vi "GD_GesamtKonz_EA_back_calc.vi"(7 "DoIt":bool, 8 "Einheit in String":string, 9 "höchste Konzentration Teilkomponente":dbl, 10 "Gesamtkonzentration":dbl, 11 "Stufentabelle (Eingang)":string[](array[string])) -> (3 "Sollwerte EA Tabelle (Ausgang)":string[](array[string]))   [LabVIEW 2020, in "Linearisierung v2.lvlib" / "Gasteiler.lvlib"]
uses:
  Gasteiler.lvlib
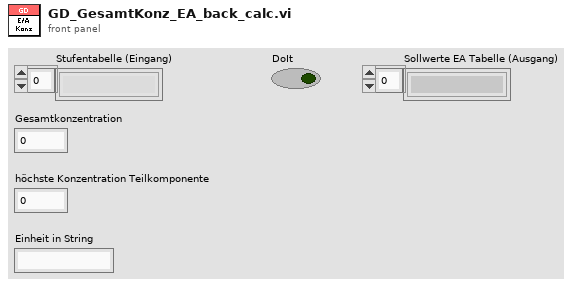
[diagram p1: front panel]
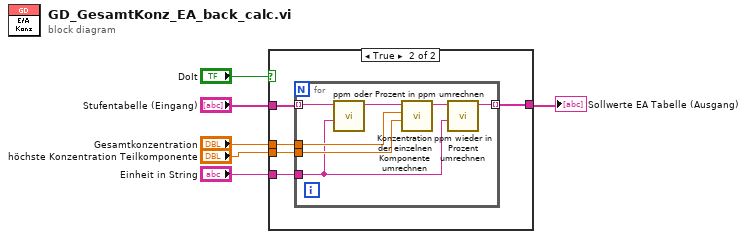
[diagram p0: block diagram]
diagram:
  n1 = case shown="True" "DoIt" {
    tunnel: "Stufentabelle (Eingang)" -> [w7 w12]
    tunnel: "Gesamtkonzentration" -> [_ w11]
    tunnel: "höchste Konzentration Teilkomponente" -> [_ w10]
    tunnel: "Einheit in String" -> [_ w9]
    tunnel: [w7 w8] -> w5
    frame False {
    }
    frame True {
      n2 = for {
        tunnel: w10 -> [w18]
        tunnel: w9 -> [w13]
        tunnel: w12 -> [w15] mode=indexing
        tunnel: w11 -> [w17]
        tunnel: [w16] -> w8 mode=indexing
        n3 = call "ppm oder Prozent in ppm umrechnen.vi"("Einheit"=w13, "Werteingang"=w15) -> ("Wertausgang"=w14:string)  [unwired: 9 in]
        n4 = call "Konzentration der einzelnen Komponente umrechnen.vi"("Teilkonzentration"=w18, "Gesamtkonzentration"=w17, "Werteingang"=w14) -> ("Wertausgang"=w19:string)  [unwired: 8 in]
        n5 = call "ppm wieder in Prozent umrechnen.vi"("Einheit"=w13, "Werteingang"=w19) -> ("Wertausgang"=w16:string)  [unwired: 9 in]
      }
    }
  }
  "Sollwerte EA Tabelle (Ausgang)" <- w5
